vi "Autonomous Independent.vi"() -> ()   [LabVIEW 2012]
doc: "This VI is called when autonomous begins, and will automatically be terminated when autonomous ends. You can carry out timed or sensor driven robot movement independently without needing to return to the caller."
uses:
  AutoInstructionCluster.ctl
  Robot Global Data.vi
  <vilib>/Rock Robotics/WPI/Joystick/WPI_JoystickGetSetRefNum.vi
  <vilib>/Rock Robotics/WPI/RobotDrive/WPI_RobotDriveArcadeDrive_Standard(NoSaturation).vi
panel:
  in  "AutoInstructions":T1[](array[typedef])
  out "Current Movement, for debugging":T2 {"Y Joystick Value" scale=1.0..-1.0; "X Joystick Value" scale=-1.0..1.0}
  in  "Array of robot movements":T3(array[cluster]) {"Y Joystick Value" scale=1.0..-1.0; "X Joystick Value" scale=-1.0..1.0}
  # "Be sure to right-click and choose Data Operations>>Make Current Value default if you want to save the array values with the VI"
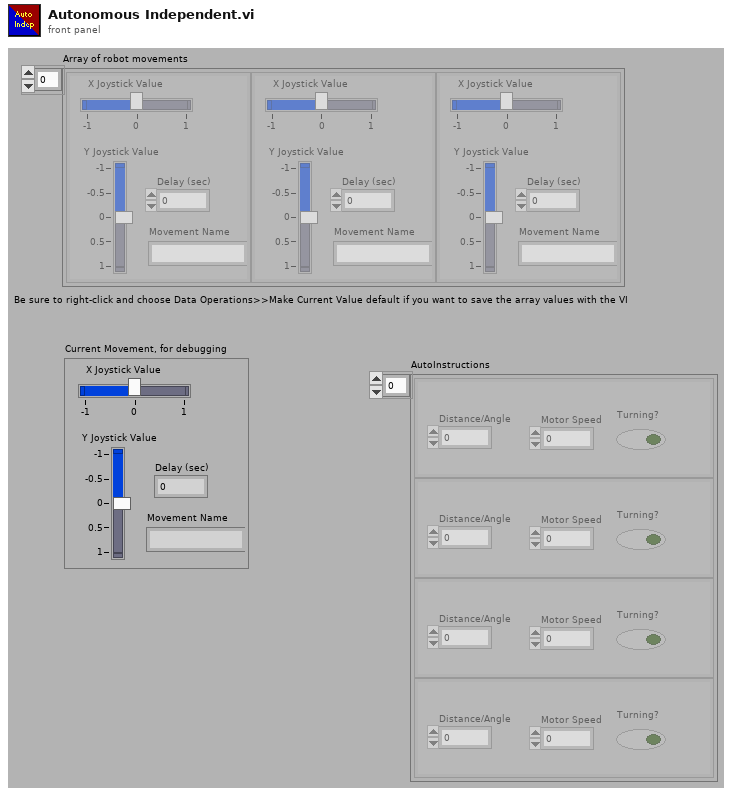
[diagram p1: front panel]
types:
  T1 = typedef "AutoInstructionCluster.ctl" = cluster{"Distance/Angle":dbl, "Motor Speed":dbl, "Turning?":bool}
  T2 = cluster{"X Joystick Value":dbl, "Y Joystick Value":dbl, "Delay (sec)":dbl, "Movement Name":string}
  T3 = cluster{"X Joystick Value":dbl, "Y Joystick Value":dbl, "Delay (sec)":dbl, "Movement Name":string}[]
  T4 = typedef "WPI_JoystickDevRef.ctl" = cluster{"Device":T5}
  T5 = typedef "WPI_JoystickDeviceEnum.ctl" = enum16{"USB 1", "USB 2", "USB 3", "USB 4", "Kinect 1", "Kinect 2"}
  T6 = cluster{"axis 1 (x)":dbl, "axis 2 (y)":dbl, "axis 3 (throttle)":dbl, "axis 4":dbl, "axis 5":dbl, "axis 6":dbl}
  T7 = typedef "WPI_RobotDriveDevRef.ctl" = cluster{"DevStatus":errorcluster, "Motors[]":T8[], "Square Inputs":bool, "Max Output":dbl, "Isochronous":bool}
  T8 = typedef "WPI_MotorControlDeviceRef.ctl" = cluster{"DeviceStatus":errorcluster, "Type":enum16{"PWM", "CAN"}, "PWM":cluster{"Digital Module":T9, "PWM Channel":T10, "DeadBand":T11}, "CAN":cluster{"Device Number":u8, "Control Mode":T12, "Semaphore":T13, "Max Vout":dbl}, "Invert":bool, "TransformRef":T14, "InvTransformRef":T14}
  T9 = typedef "FPGA_TypedefDigitalModule.ctl" = enum16{"Digital Module 1", "Digital Module 2"}
  T10 = typedef "FPGA_DIOPWMChannel.ctl" = enum8{"PWM 1", "PWM 2", "PWM 3", "PWM 4", "PWM 5", "PWM 6", "PWM 7", "PWM 8", "PWM 9", "PWM 10", "Invalid"}
  T11 = typedef "WPI_PWMDeadband.ctl" = cluster{"Name":string, "maxPositivePwm":i32, "minPositivePwm":i32, "centerPwm":i32, "maxNegativePwm":i32, "minNegativePwm":i32, "angularRange":u16}
  T12 = typedef "WPI_CANJaguar_ControlMode.ctl" = enum8{"Percent VBus", "Current", "Speed", "Position", "Voltage"}
  T13 = typedef "Semaphore RefNum" = refnum<k1>
  T14 = typedef "WPI_PWMTransform_ConPane.ctl" = refnum<vi>
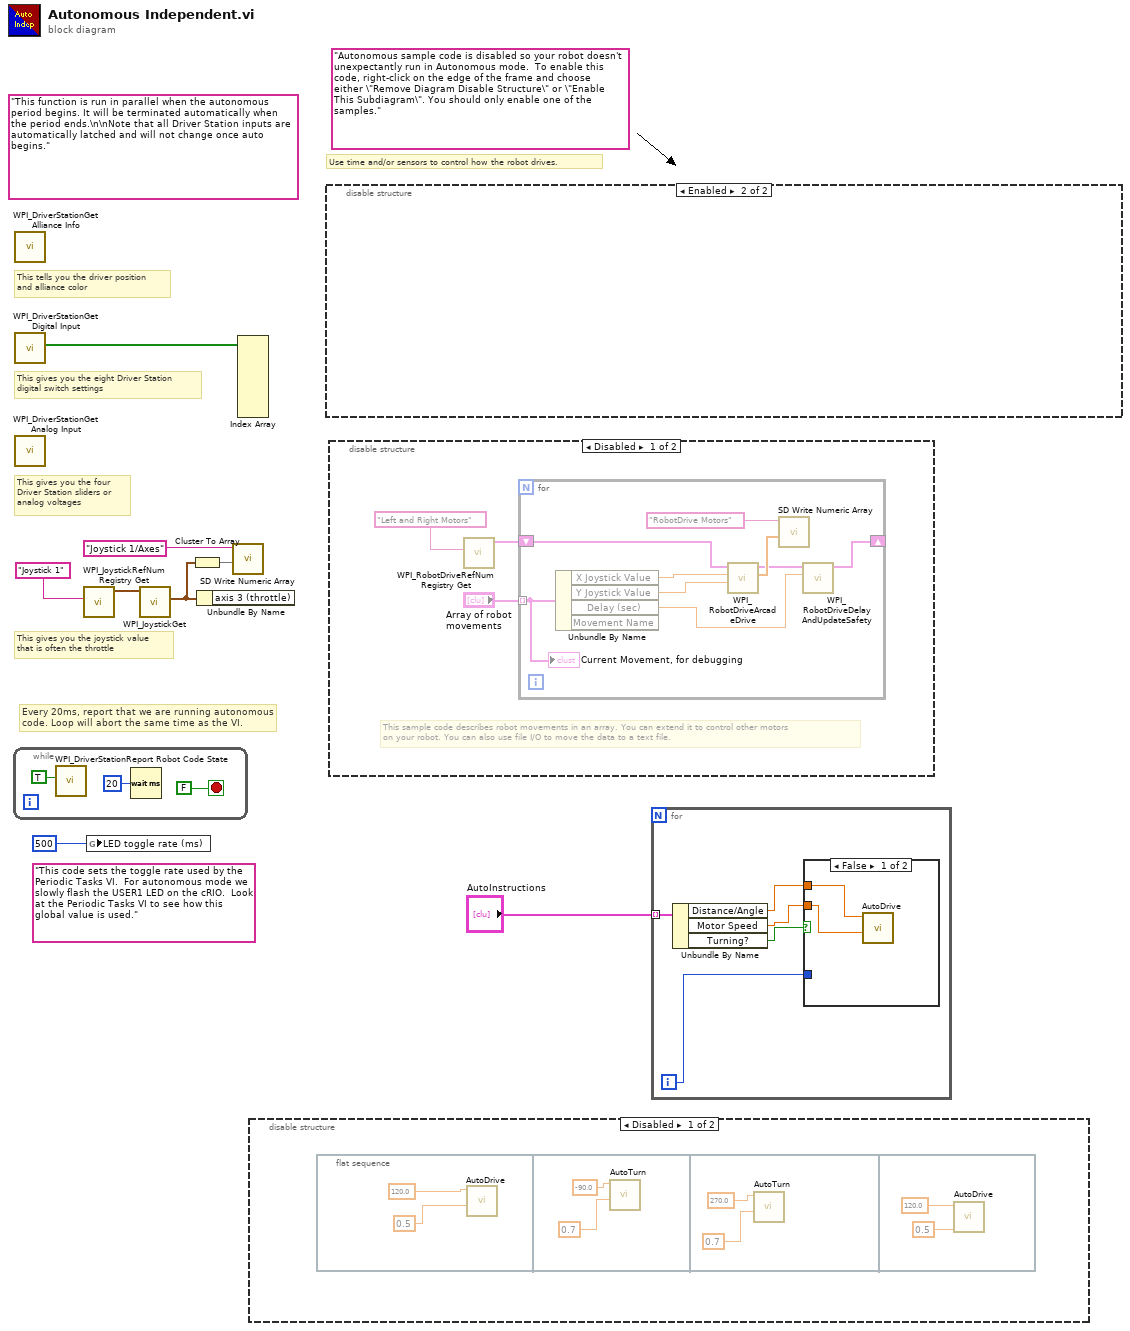
[diagram p0: block diagram]
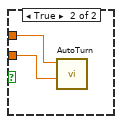
[diagram p3: hidden frame]
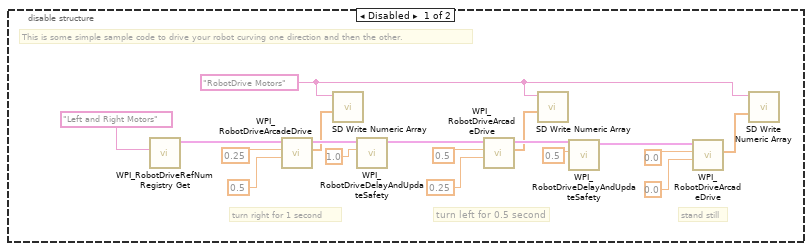
[diagram p5: hidden frame]
diagram:
  (unwired) "This code sets the toggle rate used by the Periodic Tasks VI.  For autonomous mode we slowly flash the USER1 LED on the cRIO.  Look at the Periodic Tasks VI to see how this global value is used."
  (unwired) "Autonomous sample code is disabled so your robot doesn't unexpectantly run in Autonomous mode.  To enable this code, right-click on the edge of the frame and choose either \"Remove Diagram Disable Structure\" or \"Enable This Subdiagram\". You should only enable one of the samples."
  (unwired) "This function is run in parallel when the autonomous period begins. It will be terminated automatically when the period ends.\n\nNote that all Driver Station inputs are automatically latched and will not change once auto begins."
  # "Every 20ms, report that we are running autonomous\ncode. Loop will abort the same time as the VI."
  # "This gives you the joystick value\nthat is often the throttle"
  # "Use time and/or sensors to control how the robot drives."
  # "This tells you the driver position\nand alliance color"
  # "This gives you the eight Driver Station\ndigital switch settings"
  # "This gives you the four\nDriver Station sliders or\nanalog voltages"
  n1 = while {
    stop <- FALSE stop-if-true
    n2 = call <vilib>:"WPI_DriverStationReport Robot Code State.vi"("Autonomous"=TRUE) -> ()  [unwired: 10 in, 1 out]
    n3 = Wait (ms)(milliseconds to wait=u32 20) -> ()  [unwired: 1 out]
  }
  n4 = call <vilib>:"WPI_DriverStationGet Alliance Info.vi"() -> ()  [unwired: 12 out]
  n5 = call <vilib>:"WPI_DriverStationGet Digital Input.vi"() -> ("Driver Station Digital Input (1-8)"=w8:bool[])  [unwired: 11 out]
  n6 = call <vilib>:"WPI_DriverStationGet Analog Input.vi"() -> ()  [unwired: 12 out]
  n7 = call <vilib>:"WPI_JoystickRefNum Registry Get.vi"("refnum name"="Joystick 1") -> ("JoystickDevRef"=w6:T4)  [unwired: 1 in, 9 out]
  n8 = global write "Robot Global Data.vi" "LED toggle rate (ms)"(u32 500 ("LED ms toggle rate")) -> ()
  n9 = call <vilib>:"WPI_JoystickGet.vi"("JoystickDevRef"=w6) -> ("Axes"=w3:T6)  [unwired: 1 in, 5 out]
  n10 = Cluster To Array(cluster=w3) -> (array=w4:dbl[])
  n11 = Unbundle By Name(w3) -> ()  [unwired: 1 out]
  n12 = call <vilib>:"SD Write Numeric Array.vi"("Numeric Array"=w4, "Name"="Joystick 1/Axes") -> ()  [unwired: 8 in, 2 out]
  n13 = Index Array(array=w8) -> ()  [unwired: 8 in, 8 out]
  n14 = disable-structure shown="Disabled" {
    frame Disabled {
      n15 = flat-sequence {
        frame #0 {
          n16 = call "AutoDrive.vi"("Steady Val"=0.5, "Distance to travel (inches)"=120.0) -> ()  [unwired: 10 in]
        }
        frame #1 {
          n17 = call "AutoTurn.vi"("Steady Val"=0.7, "Degrees to turn"=-90.0) -> ()  [unwired: 10 in]
        }
        frame #2 {
          n18 = call "AutoTurn.vi"("Steady Val"=0.7, "Degrees to turn"=270.0) -> ()  [unwired: 10 in]
        }
        frame #3 {
          n19 = call "AutoDrive.vi"("Steady Val"=0.5, "Distance to travel (inches)"=120.0) -> ()  [unwired: 10 in]
        }
      }
    }
    frame Enabled {
    }
  }
  n20 = disable-structure shown="Enabled" {
    frame Disabled {
      w20 = "RobotDrive Motors" ("Name")
      # "This is some simple sample code to drive your robot curving one direction and then the other."
      # "stand still"
      # "turn left for 0.5 second"
      # "turn right for 1 second"
      n21 = call <vilib>:"WPI_RobotDriveRefNum Registry Get.vi"("refnum name"="Left and Right Motors") -> ("RobotDriveDevRef"=w24:T7)  [unwired: 1 in, 9 out]
      n22 = call-poly <vilib>:"WPI_RobotDriveArcadeDrive.vi"("Y axis value"=0.5 ("X axis value"), "X axis value"=0.25, "RobotDriveDevRef"=w24) -> ("Motor Values"=w23:dbl[], "RobotDriveDevRef"=w31:T7)  [unwired: 1 in, 6 out]
      n23 = call <vilib>:"SD Write Numeric Array.vi"("Numeric Array"=w23, "Name"=w20) -> ()  [unwired: 8 in, 2 out]
      n24 = call <vilib>:"WPI_RobotDriveDelayAndUpdateSafety.vi"("Delay (s)"=1.0, "RobotDriveDevRef"=w31) -> ("RobotDriveDevRef 2"=w30:T7)  [unwired: 8 in, 1 out]
      n25 = call-poly <vilib>:"WPI_RobotDriveArcadeDrive.vi"("Y axis value"=0.25 ("X axis value"), "X axis value"=0.5, "RobotDriveDevRef"=w30) -> ("Motor Values"=w22:dbl[], "RobotDriveDevRef"=w29:T7)  [unwired: 1 in, 6 out]
      n26 = call <vilib>:"SD Write Numeric Array.vi"("Numeric Array"=w22, "Name"=w20) -> ()  [unwired: 8 in, 2 out]
      n27 = call <vilib>:"WPI_RobotDriveDelayAndUpdateSafety.vi"("Delay (s)"=0.5, "RobotDriveDevRef"=w29) -> ("RobotDriveDevRef 2"=w28:T7)  [unwired: 8 in, 1 out]
      n28 = call-poly <vilib>:"WPI_RobotDriveArcadeDrive.vi"("Y axis value"=0.0 ("X axis value"), "X axis value"=0.0, "RobotDriveDevRef"=w28) -> ("Motor Values"=w21:dbl[])  [unwired: 1 in, 7 out]
      n29 = call <vilib>:"SD Write Numeric Array.vi"("Numeric Array"=w21, "Name"=w20) -> ()  [unwired: 8 in, 2 out]
    }
    frame Enabled {
    }
  }
  n30 = disable-structure shown="Disabled" {
    frame Disabled {
      # "This sample code describes robot movements in an array. You can extend it to control other motors\non your robot. You can also use file I/O to move the data to a text file."
      n31 = call <vilib>:"WPI_RobotDriveRefNum Registry Get.vi"("refnum name"="Left and Right Motors") -> ("RobotDriveDevRef"=w39:T7)  [unwired: 1 in, 9 out]
      n32 = for {
        shift-right: [w45] -> _
        shift-left: w39 -> [w46]
        tunnel: "Array of robot movements" -> [w41] mode=indexing
        n33 = Unbundle By Name(w41) -> ("X Joystick Value"=w44:dbl, "Y Joystick Value"=w43:dbl, "Delay (sec)"=w42:dbl)  [unwired: 1 out]
        n34 = call-poly <vilib>:"WPI_RobotDriveArcadeDrive.vi"("Y axis value"=w43, "X axis value"=w44, "RobotDriveDevRef"=w46) -> ("Motor Values"=w48:dbl[], "RobotDriveDevRef"=w47:T7)  [unwired: 1 in, 6 out]
        n35 = call <vilib>:"SD Write Numeric Array.vi"("Numeric Array"=w48, "Name"="RobotDrive Motors") -> ()  [unwired: 8 in, 2 out]
        n36 = call <vilib>:"WPI_RobotDriveDelayAndUpdateSafety.vi"("Delay (s)"=w42, "RobotDriveDevRef"=w47) -> ("RobotDriveDevRef 2"=w45:T7)  [unwired: 8 in, 1 out]
        "Current Movement, for debugging" <- w41
      }
    }
    frame Enabled {
    }
  }
  n37 = for {
    tunnel: "AutoInstructions" -> [w54] mode=indexing
    i -> [w50]
    n38 = Unbundle By Name(w54) -> ("Distance/Angle"=w52:dbl, "Motor Speed"=w51:dbl, "Turning?"=w53:bool)
    n39 = case shown="False" w53 {
      tunnel: w52 -> [w56 w58]
      tunnel: w51 -> [w55 w57]
      tunnel: w50 -> [_ _]
      frame False {
        n40 = call "AutoDrive.vi"("Steady Val"=w55, "Distance to travel (inches)"=w56) -> ()  [unwired: 10 in]
      }
      frame True {
        n41 = call "AutoTurn.vi"("Steady Val"=w57, "Degrees to turn"=w58) -> ()  [unwired: 10 in]
      }
    }
  }
